vi "Make Bent Wire Straight.vi"(8 "error in (no error)":errorcluster, 10 "Index (-1 For All)":i32=-1, 11 "CSM-Helper In":refnum<class "CSM-Helper.lvclass">) -> (0 "error out":errorcluster, 3 "CSM-Helper Out":refnum<class "CSM-Helper.lvclass">)   [LabVIEW 2017, in "CSM-Helper.lvclass"]
uses:
  CSM-Helper.lvclass
  Utility/_Support/PairedTunnels.llb/csmHelper-PairedTunnels.lvlib
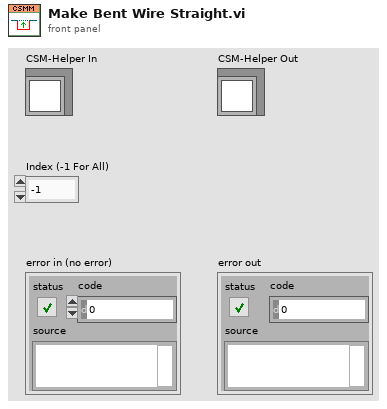
[diagram p1: front panel]
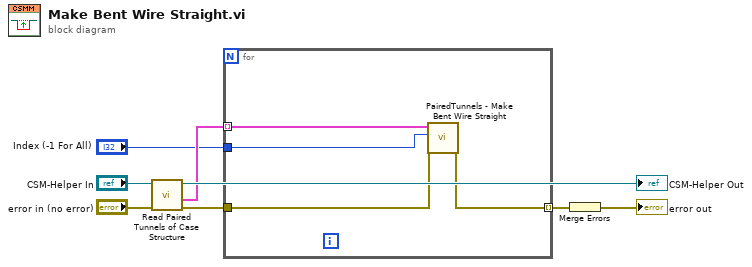
[diagram p0: block diagram]
diagram:
  n1 = call "Read Paired Tunnels of Case Structure.vi"("error in (no error)"="error in (no error)", "CSM-Helper in"="CSM-Helper In") -> ("error out"=w3:errorcluster, "Paired Tunnels"=w4:cluster{refnum<vi>, refnum<vi>}[], "CSM-Helper out"=→"CSM-Helper Out":refnum<class "CSM-Helper.lvclass">)  [unwired: 7 in]
  n2 = for {
    tunnel: w4 -> [w12] mode=indexing
    tunnel: w3 -> [w11]
    tunnel: [w10] -> w5 mode=indexing
    tunnel: "Index (-1 For All)" -> [w9]
    n3 = call "PairedTunnels - Make Bent Wire Straight.vi"("Error in"=w11, "index(-1 for all)"=w9, "PairedTunnels"=w12) -> ("error out"=w10:errorcluster)  [unwired: 7 in, 1 out]
  }
  n4 = Merge Errors(w5) -> (→"error out":errorcluster)
